vi "Uint64 Create.vi"(8 "error in (no error)":errorcluster, 11 "U64 in":u64) -> (0 "error out":errorcluster, 3 "Uint64 DVR out":refnum<data-value>)   [LabVIEW 2012, in "MDSplus.lvlib"]
uses:
  <vilib>/MDSplus/Library/MDSplus.lvlib
  <vilib>/MDSplus/Classes/Data_Class/Scalar_Class/Uint64_Class/Uint64.lvclass
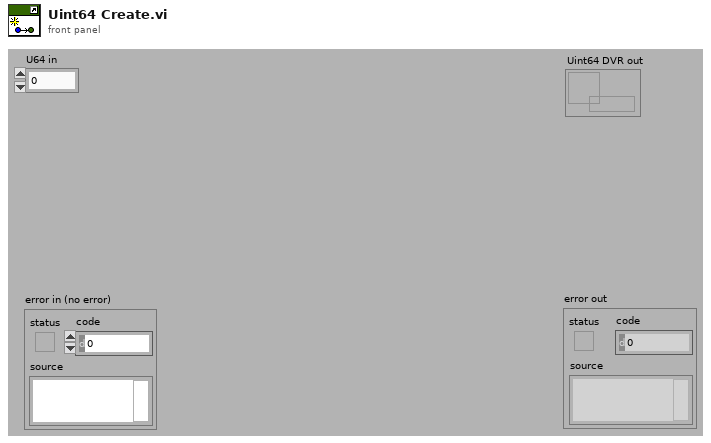
[diagram p1: front panel]
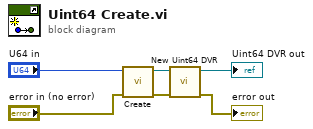
[diagram p0: block diagram]
diagram:
  n1 = call <vilib>:"Create.vi"("error in (no error)"="error in (no error)", "U64 in"="U64 in") -> ("error out"=w3:errorcluster, "Uint64 out"=w4:refnum<class "Uint64.lvclass">)  [unwired: 8 in]
  n2 = call <vilib>:"New Uint64 DVR.vi"("error in (no error)"=w3, "Uint64 in"=w4) -> ("error out"=→"error out":errorcluster, "Uint64 DVR out"=→"Uint64 DVR out":refnum<data-value>)  [unwired: 8 in]
